vi "imp_test_v11_p3.vi"() -> ()   [LabVIEW 2014]
uses:
  <vilib>/LabVIEW Targets/FPGA/cRIO/shared/nicrio_ModuleControls/nicrio_cRIO-9237_DataRatesRing.ctl
  <vilib>/LabVIEW Targets/FPGA/cRIO/shared/nicrio_ModuleControls/nicrio_cRIO-9237_ExcitationVoltageRing.ctl
  <vilib>/rvi/FXPMathLib/FxpSinAndCos/subVIs/nifxpmath_SinAndCos_SimConfig.ctl
  <vilib>/rvi/Emulation/niFpgaGetClockAttributes.vi
  <vilib>/rvi/Emulation/niFpgaSctlEmulationGetInTimedLoop.vi
  <vilib>/rvi/Emulation/niFpgaEmulationReportErrorSimple.vi
  <vilib>/rvi/Emulation/niFpgaProcessEmulError.vi
  <vilib>/rvi/interface/RandomDataEmulation/nirviRandomDataMultiElementFPGAFIFO.vi
  <instcachedir>/0/nirviRandomDataMultiElementFPGAFIFO_AD0CFC12EF974623A9C2E4184BC062B2.lvgen/nirviRandomDataMultiElementFPGAFIFO_AD0CFC12EF974623A9C2E4184BC062B2_028.vi
  <vilib>/rvi/interface/RandomDataEmulation/niFpgaRandomDataHandleErrors.vi
  <vilib>/rvi/Emulation/niFpgaCriticalErrorInLSC.vi
  <vilib>/rvi/FXPMathLib/FxpSinAndCos/simVIs/DllFxpSinAndCosTemp_sub.vi
  <vilib>/rvi/eio/common/nirviEmuTemplateMethod_errors.vi
  <vilib>/rvi/eio/common/nirviEmuTemplatePropertySet_errors.vi
  <vilib>/rvi/DataTransferAndStorage/Container/XNode/niFpgaContainer.xnode
  <vilib>/rvi/interface/RandomDataEmulation/nirviRandomDataFpgaMultiElementTemplate.vi
  <vilib>/rvi/Analysis/measure/butterworth/XNode/niFpgaButterworthFilter.xnode
  <vilib>/rvi/FXPMathLib/FxpSinAndCos/XNode/nifxpmath_SinAndCos.xnode
  <vilib>/eio/EIONode/EIONode.xnode
  <vilib>/eio/EIOPropertyNode/EIOPropertyNode.xnode
  <vilib>/rvi/eio/common/nirviEmuTemplatePropertyGet_errors.vi
  <vilib>/rvi/eio/common/nirviEmuTemplatePropertyGet_noerrors.vi
  <vilib>/rvi/eio/common/nirviEmuTemplatePropertySet_noerrors.vi
panel:
  in  "force_lim":fxp<+,22,9>
  in  "Mavg f loop(uSec)":u32
  in  "F_Threshold_p":fxp<+,12,4>
  out "omega_p (Mavg)":fxp<+/-,36,13>
  out "Dp_d (Mavg)":fxp<+/-,36,13>
  out "omega_p2 (Mavg)":fxp<+/-,36,14>
  out "Dp2_d (Mavg)":fxp<+/-,36,14>
  in  "mt0_p2":u32
  out "Dp_d (Mavg w. f.)":fxp<+/-,36,14>
  in  "Dp_d (Mavg) coeff.":i32[](array[numeric])=[946630756, 63555534]
  out "omega_p (Mavg w. f)":fxp<+/-,36,14>
  in  "omega_P(Mavg) coeff.":i32[](array[numeric])=[946630756, 63555534]
  out "PID (kHz)":fxp<+/-,20,10>
  in  "Set 6":bool
  in  "Set 5":bool
  in  "Set 4":bool
  in  "Set 3":bool
  in  "Set 2":bool
  in  "Set 1":bool
  out "Dp1_d (T)":fxp<+/-,36,13>
  out "omega_p1 (T)":fxp<+/-,36,13>
  out "Dp2_d (T)":fxp<+/-,36,13>
  out "omega_p2 (T)":fxp<+/-,36,13>
  out "mt_omega_p2":u32
  out "Encoder Position_p2":i32
  out "D_p2":fxp<+/-,32,7>
  out "rad_p2":fxp<+/-,33,20>
  out "D_p1":fxp<+/-,32,7>
  out "rad_p1":fxp<+/-,33,20>
  out "Encoder Position_p1":i32
  out "Dp1_d (Mavg)":fxp<+/-,36,14>
  out "omega_p1 (Mavg)":fxp<+/-,36,14>
  in  "Dp_d_M_avg_Tc (uSec)":i32
  out "Dp_d (T)":fxp<+/-,36,13>
  out "omega_p (T)":fxp<+/-,36,13>
  in  "Vp. Est.":i16(ring) items=["T", "Mavg", "Mavg w. f."]
  in  "Mag. factor_p":fxp<+/-,20,3>
  in  "Mag. encoder_p":bool
  in  "Belt_out_p":fxp<+/-,7,7>
  in  "Belt_in_p":fxp<+/-,6,6>
  out "Fp_dc":fxp<+/-,32,10>
  in  "Zero_p":bool
  in  "mt0_p1":u32
  in  "Encoder reset":bool
  out "fpt_d":fxp<+/-,36,18>
  out "Dp_error_dd":fxp<+/-,36,16>
  out "Dp_error_d":fxp<+/-,33,8>
  in  "Dp_dd coeff.":i32[](array[numeric])=[946630756, 63555534]
  out "Dp_dd":fxp<+/-,36,25>
  out "dFp_PID":fxp<+/-,36,18>
  in  "dFp_PID coeff.":i32[](array[numeric])=[946630756, 63555534]
  out "fpt_i":fxp<+/-,34,18>
  in  "Bv_p":fxp<+/-,22,8>
  in  "Kv_p":fxp<+/-,26,7>
  out "Dp_error":fxp<+/-,22,7>
  out "Dpr_sin":fxp<+/-,22,7>
  in  "Sin offset_p":fxp<+/-,22,7>
  in  "Sin magnitude_p":fxp<+/-,21,6>
  out "Dpr_sin_dd":fxp<+/-,35,20>
  out "Dpr_sin_d":fxp<+/-,33,15>
  out "Sin omega_p":fxp<+/-,34,9>
  in  "Sin wave freq._p (Hz)":fxp<+/-,32,6>
  in  "Dpr_step":fxp<+/-,22,7>
  out "Dpr_for":fxp<+/-,22,7>
  in  "Command_p":i16(ring) items=["Step", "Sine"]
  in  "Ki_p":fxp<+/-,30,9>
  out "Fp_PID":fxp<+/-,36,16>
  in  "fp_tolorance":fxp<+,22,6>
  out "fp_tilde":fxp<+/-,33,10>
  in  "Kd_p":fxp<+/-,30,9>
  in  "Kp_p":fxp<+/-,32,13>
  out "Fr_p":fxp<+/-,32,10>
  in  "S/F coeff_p":fxp<+/-,25,-10>
  out "va_p":fxp<+/-,36,7>
  out "vb_p":fxp<+/-,37,8>
  out "vq_p_F":fxp<+/-,20,5> format="%.57g"
  out "vd_p_F":fxp<+/-,20,5>
  in  "dFp_add":bool
  in  "Stop motor_p":bool
  out "Force_p":fxp<+/-,32,10>
  in  "Strain selection_p":i16(ring) items=["Raw", "Avg.8", "Avg.8 w. filter"]
  out "Strain_p (Avg8 w. f)":fxp<+/-,36,8>
  in  "Strain_p Avg.8 coeff.":i32[](array[numeric])=[946630756, 63555534]
  out "Strain_p (Avg8)":fxp<+/-,36,4>
  out "Raw Strain_p":fxp<+/-,36,4>
  out "Mod6/AI3":fxp<+/-,36,4>
  in  "Strain gage reset_p":bool
  out "Dp_d (mm/s)":fxp<+/-,36,13>
  out "omega_p (rad/s)":fxp<+/-,36,13>
  out "mt_omega_p1":u32
  out "rad_p(NrTheta)":fxp<+/-,33,20>
  out "D_p(mm)":fxp<+/-,32,7>
  out "Encoder Position_p":i32
  in  "Encoder reset_p":bool
  out "Time now(s)":fxp<+,52,14>
  in  "Drive mode":i16(ring) items=["Backward", "Forward", "Imp"]
  in  "Ini coe.":bool
  out "Loop rate (kHz)":fxp<+/-,36,7>
  in  "Stop (Strain)":bool
  in  "Excitation Voltage":T1 items=["2.5 Volts", "3.3 Volts", "5.0 Volts", "10.0 Volts", "External Excitation"]
  in  "Data Rate":T2=1 items=["50.000 kS/s (NI 9237)"=1, "25.000 kS/s (NI 9237)"=2, "16.667 kS/s (NI 9237)"=3, "12.500 kS/s (NI 9237)"=4, "10.000 kS/s (NI 9237)"=5, "8.333 kS/s (NI 9237)"=6, "7.143 kS/s (NI 9237)"=7, "6.250 kS/s (NI 9237)"=8, "5.556 kS/s (NI 9237)"=9, "5.000 kS/s (NI 9237)"=10, "4.545 kS/s (NI 9237)"=11, "4.167 kS/s (NI 9237)"=12, "3.846 kS/s (NI 9237)"=13, "3.571 kS/s (NI 9237)"=14, "3.333 kS/s (NI 9237)"=15, "3.125 kS/s (NI 9237)"=16, "2.941 kS/s (NI 9237)"=17, "2.778 kS/s (NI 9237)"=18, "2.632 kS/s (NI 9237)"=19, "2.500 kS/s (NI 9237)"=20, "2.381 kS/s (NI 9237)"=21, "2.273 kS/s (NI 9237)"=22, "2.174 kS/s (NI 9237)"=23, "2.083 kS/s (NI 9237)"=24, "2.000 kS/s (NI 9237)"=25, "1.923 kS/s (NI 9237)"=26, "1.852 kS/s (NI 9237)"=27, "1.786 kS/s (NI 9237)"=28, "1.724 kS/s (NI 9237)"=29, "1.667 kS/s (NI 9237)"=30, "1.613 kS/s (NI 9237)"=31]
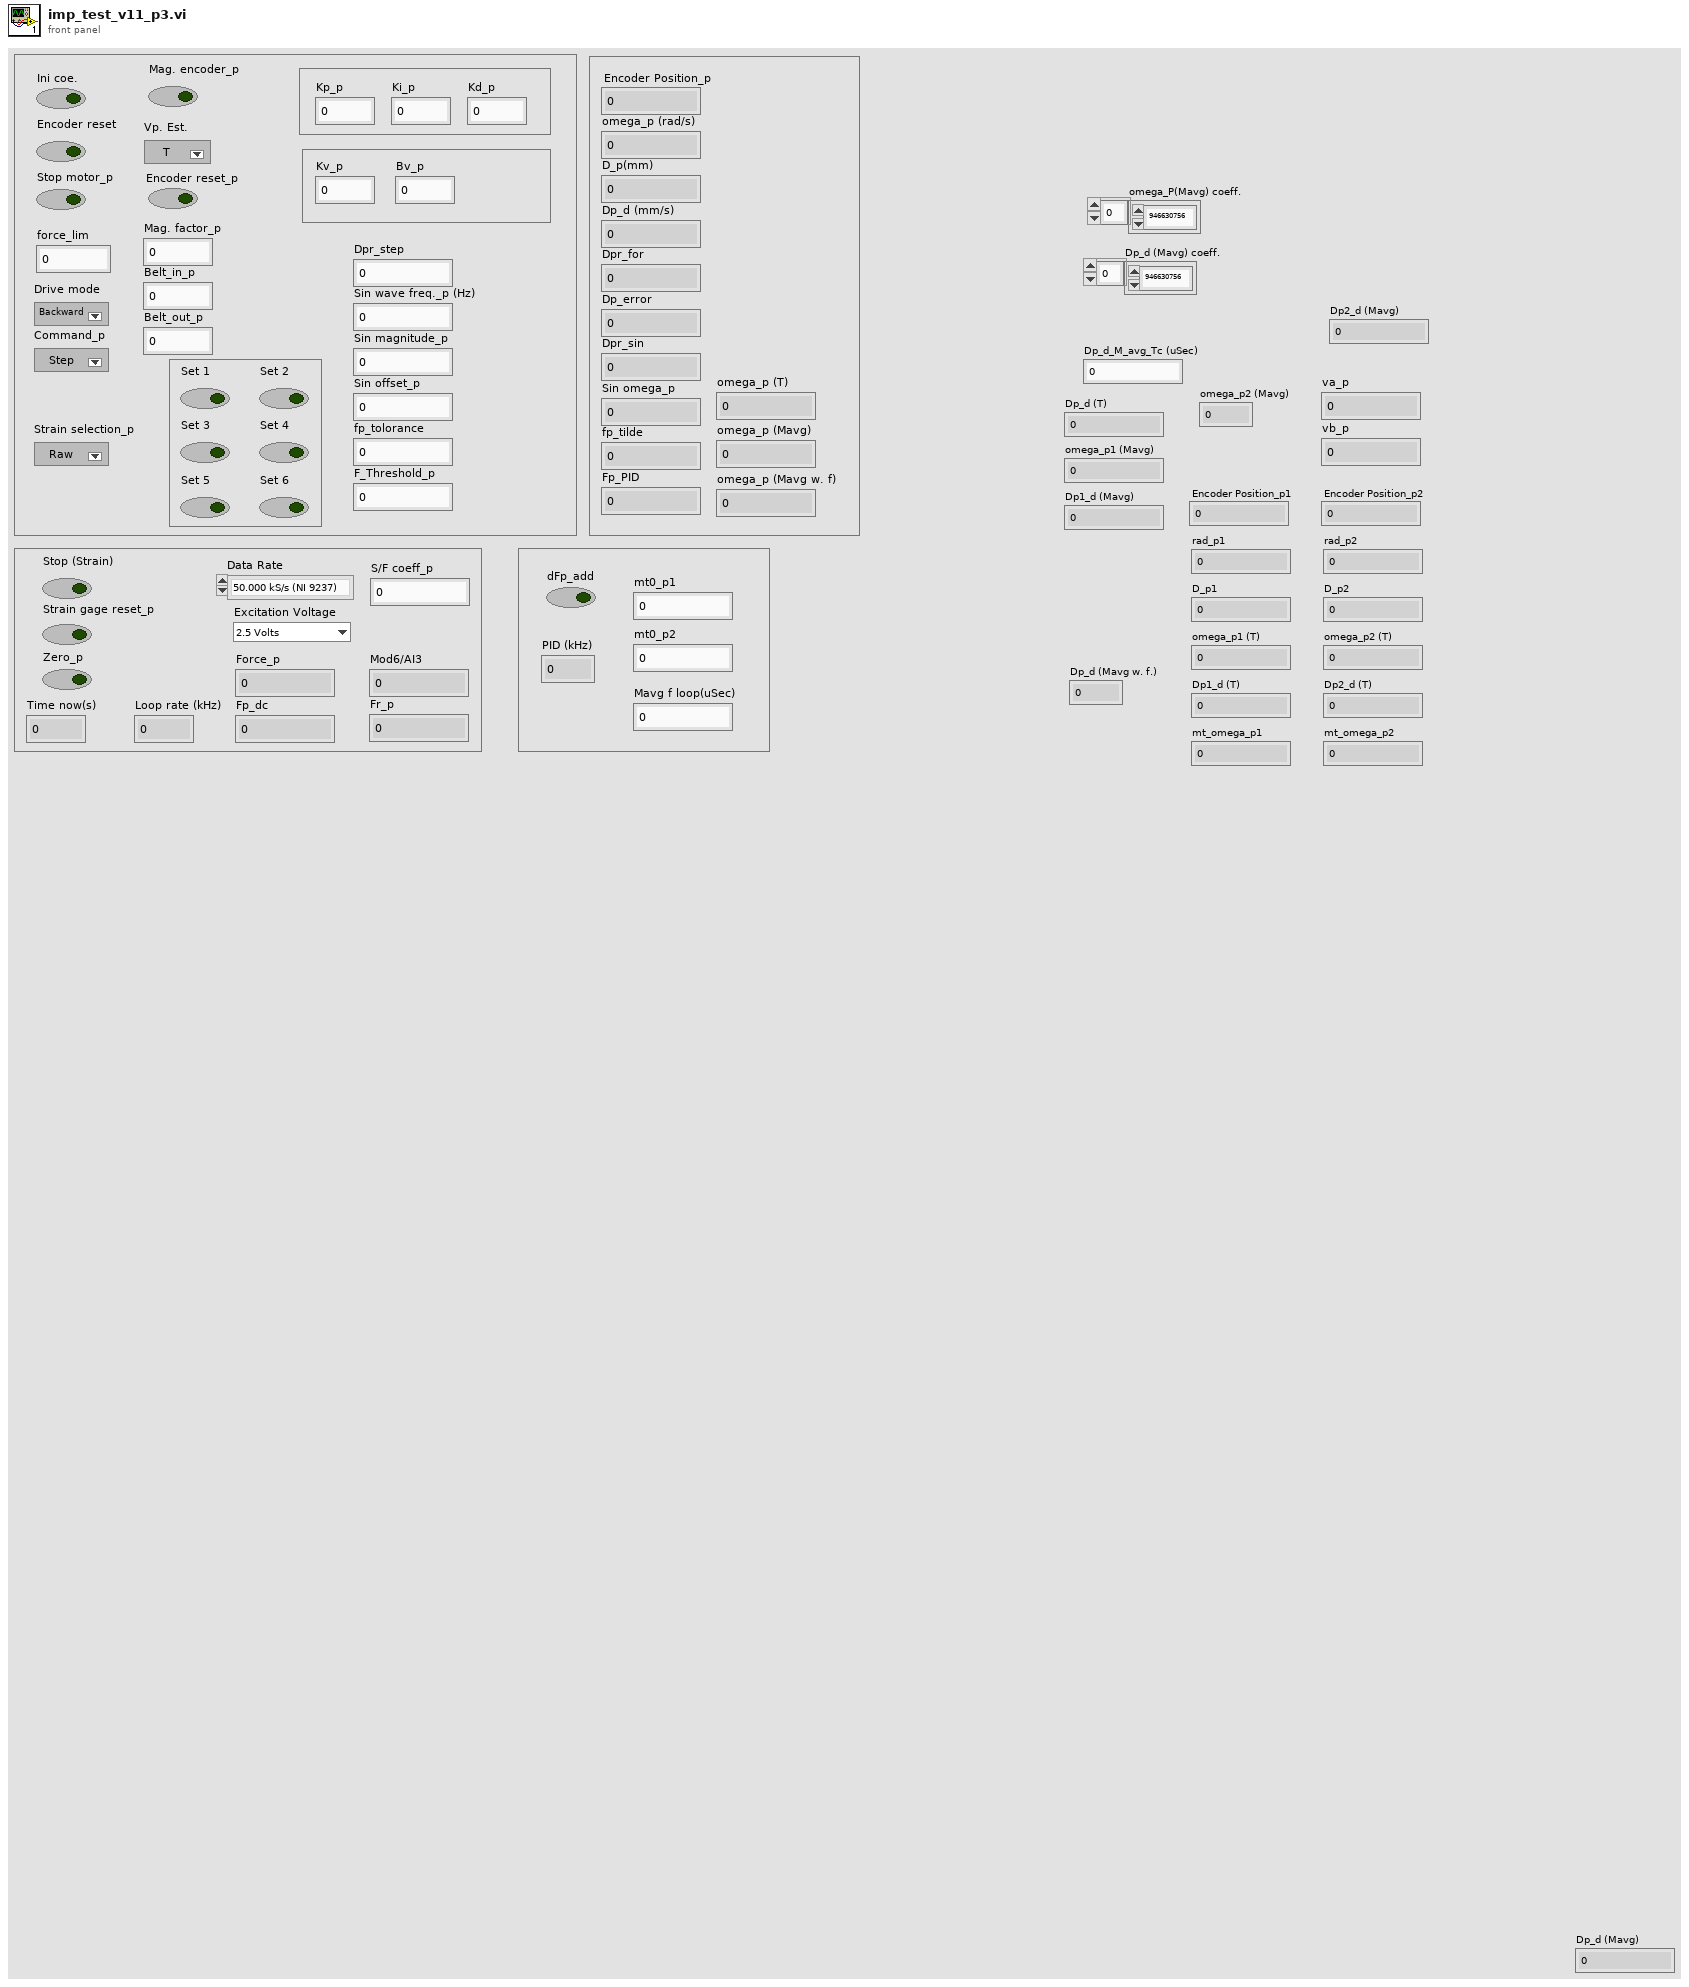
[diagram p1: front panel]
types:
  T1 = typedef "nicrio_cRIO-9237_ExcitationVoltageRing.ctl" = u8
  T2 = typedef "nicrio_cRIO-9237_DataRatesRing.ctl" = u8
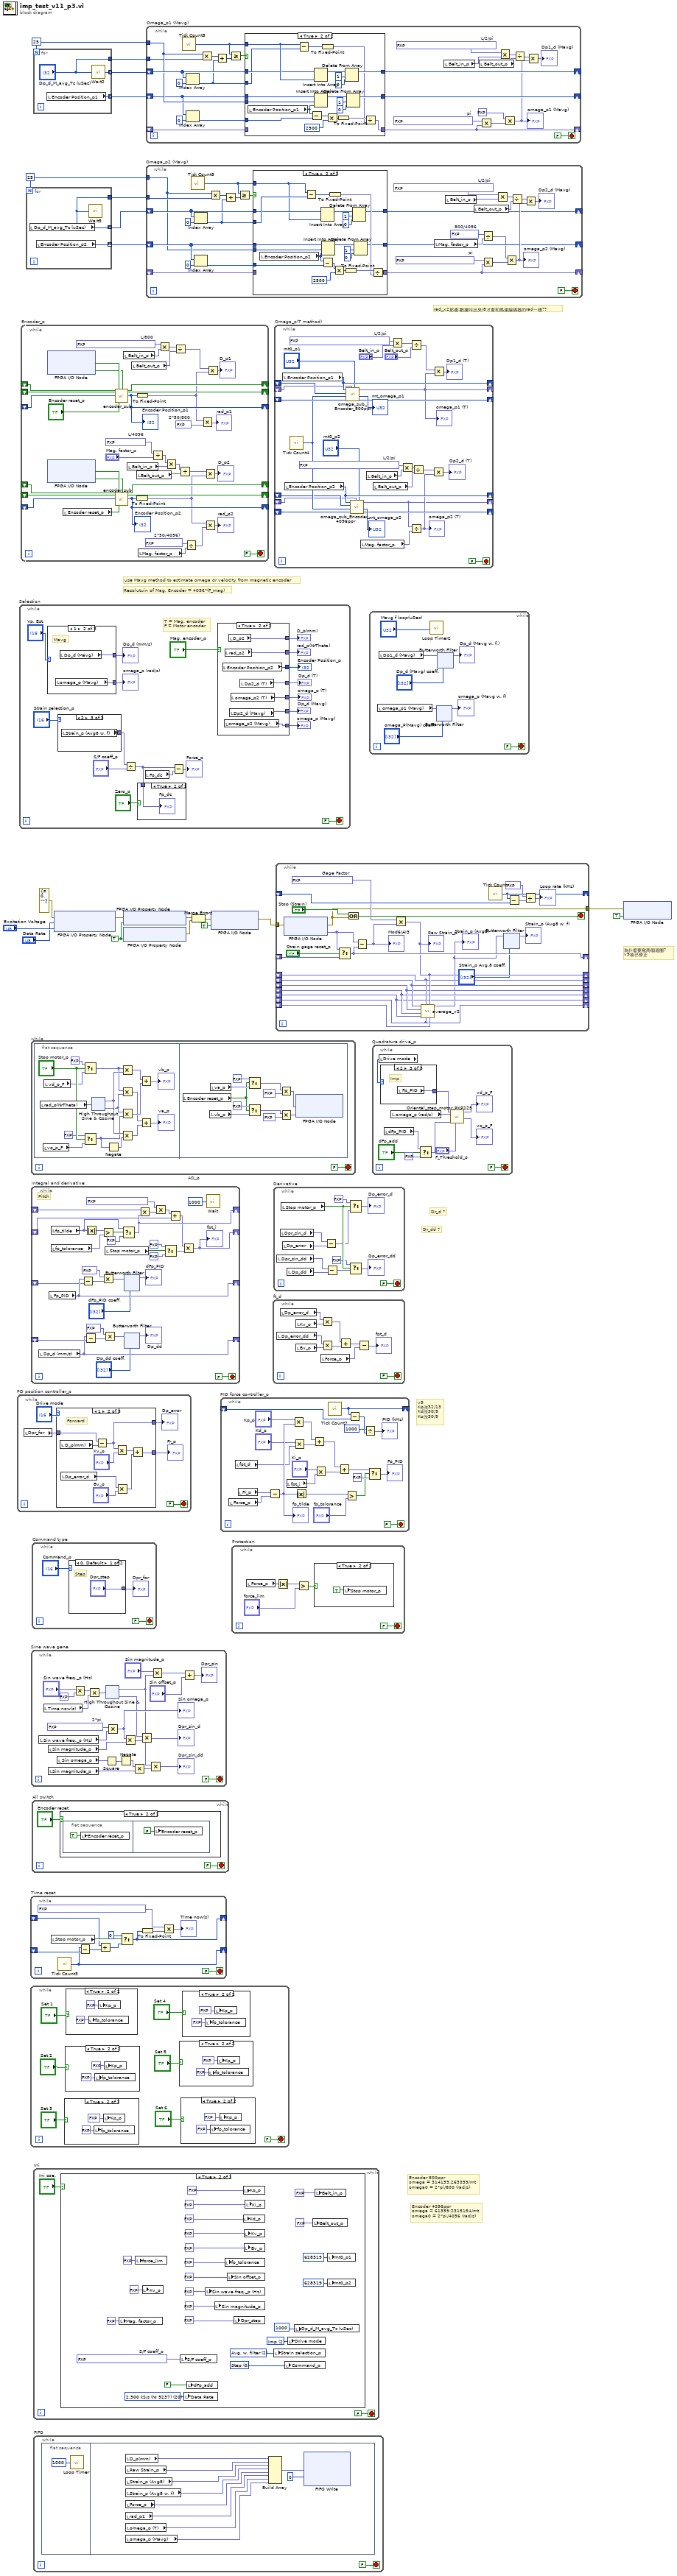
[diagram p0: block diagram]
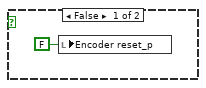
[diagram p11: hidden frame]
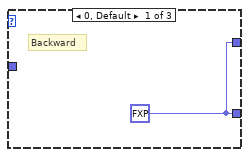
[diagram p12: hidden frame]
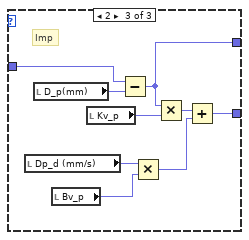
[diagram p13: hidden frame]
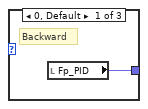
[diagram p14: hidden frame]
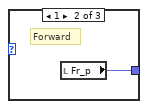
[diagram p15: hidden frame]
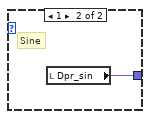
[diagram p16: hidden frame]
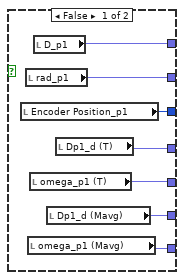
[diagram p17: hidden frame]
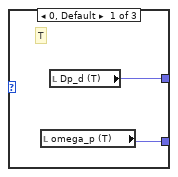
[diagram p18: hidden frame]
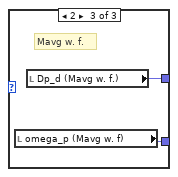
[diagram p19: hidden frame]
diagram:
  w2 = 25
  w8 = 25
  w13 = TRUE ("Half-Bridge Enable")
  # "rad_x2那邊:數據叫出來/8才會和馬達編碼器的rad一樣??"
  # "Encoder 4096ppr\nomega = 61359.2315154/mt\nomega0 = 2*pi/4096 (rad/s)"
  # "Encoder 800ppr\nomega = 314159.265359/mt\nomega0 = 2*pi/800 (rad/s)"
  # "v9\nKp改32/13\nKd改30/9\nKo改30/9"
  # "Resolutuin of Mag. Encoder = 4096*(F_mag)"
  # "use Mavg method to estimate omega or velocity from magnetic encoder"
  # "為什麼要寫兩個迴圈?\nv9後已修正"
  # "Dr_dd ?"
  # "Dr_d ?"
  n1 = while "PD position controller_p" {
    stop <- FALSE stop-if-true
    n2 = local read "Dpr_for"() -> (w21:fxp<+/-,22,7>)
    n3 = case shown="1" "Drive mode" {
      tunnel: [w26 w30 w37] -> w25
      tunnel: [w26 w28 w42] -> w22
      tunnel: w21 -> [_ w27 w36]
      frame 0, Default {
        w26 = fxp<+/-,62,19> 0.0
        # "Backward"
      }
      frame 1 {
        # "Forward"
        n4 = local read "D_p(mm)"() -> (w35:fxp<+/-,32,7>)
        n5 = local read "Dp_error_d"() -> (w29:fxp<+/-,33,8>)
        n6 = Subtract(x=w27, y=w35) -> (x-y=w28:fxp<+/-,33,8>)
        n7 = Multiply(x=w28, y="Kv_p") -> (x*y=w32:fxp<+/-,58,14>)
        n8 = Multiply(x=w29, y="Bv_p") -> (x*y=w31:fxp<+/-,55,16>)
        n9 = Add(x=w32, y=w31) -> (x+y=w30:fxp<+/-,60,16>)
      }
      frame 2 {
        # "Imp"
        n10 = local read "Dp_d (mm/s)"() -> (w40:fxp<+/-,36,13>)
        n11 = local read "D_p(mm)"() -> (w43:fxp<+/-,32,7>)
        n12 = local read "Bv_p"() -> (w39:fxp<+/-,22,8>)
        n13 = local read "Kv_p"() -> (w44:fxp<+/-,26,7>)
        n14 = Subtract(x=w36, y=w43) -> (x-y=w42:fxp<+/-,33,8>)
        n15 = Multiply(x=w40, y=w39) -> (x*y=w38:fxp<+/-,58,21>)
        n16 = Multiply(x=w42, y=w44) -> (x*y=w41:fxp<+/-,58,14>)
        n17 = Add(x=w41, y=w38) -> (x+y=w37:fxp<+/-,64,21>)
      }
    }
    "Fr_p" <- w25
    "Dp_error" <- w22
  }
  n18 = while "Selection" {
    stop <- FALSE stop-if-true
    # "T = Mag. encoder\nF = Motor encoder"
    n19 = case shown="1" "Vp. Est." {
      tunnel: [w79 w80 w83] -> w55
      tunnel: [w78 w81 w82] -> w56
      frame 0, Default {
        # "T"
        n20 = local read "omega_p (T)"() -> (w79:fxp<+/-,36,13>)
        n21 = local read "Dp_d (T)"() -> (w78:fxp<+/-,36,13>)
      }
      frame 1 {
        # "Mavg"
        n22 = local read "omega_p (Mavg)"() -> (w80:fxp<+/-,36,13>)
        n23 = local read "Dp_d (Mavg)"() -> (w81:fxp<+/-,36,13>)
      }
      frame 2 {
        # "Mavg w. f."
        n24 = local read "omega_p (Mavg w. f)"() -> (w83:fxp<+/-,36,14>)
        n25 = local read "Dp_d (Mavg w. f.)"() -> (w82:fxp<+/-,36,14>)
      }
    }
    "Dp_d (mm/s)" <- w56
    "omega_p (rad/s)" <- w55
    n26 = case shown="2" "Strain selection_p" {
      tunnel: [w85 w86 w87] -> w62
      frame 0, Default {
        n27 = local read "Raw Strain_p"() -> (w85:fxp<+/-,36,4>)
      }
      frame 1 {
        n28 = local read "Strain_p (Avg8)"() -> (w86:fxp<+/-,36,4>)
      }
      frame 2 {
        n29 = local read "Strain_p (Avg8 w. f)"() -> (w87:fxp<+/-,36,8>)
      }
    }
    n30 = Divide(x=w62, y="S/F coeff_p") -> (x/y=w59:fxp<+/-,32,10>)
    n31 = case shown="True" "Zero_p" {
      tunnel: w59 -> [_ w84]
      frame False {
      }
      frame True {
        "Fp_dc" <- w84
      }
    }
    n32 = local read "Fp_dc"() -> (w57:fxp<+/-,32,10>)
    n33 = Subtract(x=w59, y=w57) -> (x-y=→"Force_p":fxp<+/-,33,11>)
    n34 = case shown="True" "Mag. encoder_p" {
      tunnel: [w70 w77] -> w51
      tunnel: [w69 w76] -> w52
      tunnel: [w68 w75] -> w53
      tunnel: [w66 w74] -> w49
      tunnel: [w67 w73] -> w48
      tunnel: [w65 w71] -> w47
      tunnel: [w64 w72] -> w46
      frame False {
        n35 = local read "Encoder Position_p1"() -> (w68:i32)
        n36 = local read "rad_p1"() -> (w69:fxp<+/-,33,20>)
        n37 = local read "omega_p1 (Mavg)"() -> (w64:fxp<+/-,36,14>)
        n38 = local read "omega_p1 (T)"() -> (w66:fxp<+/-,36,13>)
        n39 = local read "D_p1"() -> (w70:fxp<+/-,32,7>)
        n40 = local read "Dp1_d (Mavg)"() -> (w65:fxp<+/-,36,14>)
        n41 = local read "Dp1_d (T)"() -> (w67:fxp<+/-,36,13>)
      }
      frame True {
        n42 = local read "Encoder Position_p2"() -> (w75:i32)
        n43 = local read "omega_p2 (Mavg)"() -> (w72:fxp<+/-,36,14>)
        n44 = local read "rad_p2"() -> (w76:fxp<+/-,33,20>)
        n45 = local read "D_p2"() -> (w77:fxp<+/-,32,7>)
        n46 = local read "Dp2_d (Mavg)"() -> (w71:fxp<+/-,36,14>)
        n47 = local read "omega_p2 (T)"() -> (w74:fxp<+/-,36,13>)
        n48 = local read "Dp2_d (T)"() -> (w73:fxp<+/-,36,13>)
      }
    }
    "D_p(mm)" <- w51
    "rad_p(NrTheta)" <- w52
    "Encoder Position_p" <- w53
    "Dp_d (T)" <- w48
    "omega_p (T)" <- w49
    "Dp_d (Mavg)" <- w47
    "omega_p (Mavg)" <- w46
  }
  n49 = while "Encoder_p" {
    shift-right: [w125] -> _
    shift-left: _ -> [w124]
    shift-right: [w126] -> _
    shift-left: _ -> [w123]
    shift-right: [w120] -> _
    shift-left: _ -> [w122]
    shift-right: [w111] -> _
    shift-left: _ -> [w110]
    shift-right: [w112] -> _
    shift-left: _ -> [w113]
    shift-right: [w107] -> _
    shift-left: _ -> [w108]
    stop <- FALSE stop-if-true
    w103 = fxp<+/-,20,-5> 0.00048828125  # L/4096
    w101 = fxp<+/-,16,1> 0.0244140625  # 2*50/4096)
    w119 = fxp<+/-,20,-5> 0.002499997615814209  # L/800
    w93 = fxp<+/-,16,1> 0.125  # 2*50/800
    n50 = xnode "FPGA I/O Node"() -> ("Mod7/DIO0"=w128:bool, "Mod7/DIO1"=w127:bool)  [unwired: 2 in, 2 out]
    n51 = xnode "FPGA I/O Node"() -> ("Mod7/DIO4"=w115:bool, "Mod7/DIO5"=w114:bool)  [unwired: 2 in, 2 out]
    n52 = local read "Encoder reset_p"() -> (w109:bool)
    n53 = call "encoder_sub.vi"("A_pre"=w124, "B_pre"=w123, "Encoder Position_pre"=w122, "A input"=w128, "Encoder Position Reset"="Encoder reset_p", "B input"=w127) -> ("A"=w125:bool, "B"=w126:bool, "Encoder Position (Counts)"=w120:i32)  [unwired: 19 in]
    "Encoder Position_p1" <- w120
    n54 = call "encoder_sub.vi"("A_pre"=w110, "B_pre"=w113, "Encoder Position_pre"=w108, "A input"=w115, "Encoder Position Reset"=w109, "B input"=w114) -> ("A"=w111:bool, "B"=w112:bool, "Encoder Position (Counts)"=w107:i32)  [unwired: 19 in]
    "Encoder Position_p2" <- w107
    n55 = local read "Belt_in_p"() -> (w118:fxp<+/-,6,6>)
    n56 = local read "Belt_in_p"() -> (w104:fxp<+/-,6,6>)
    n57 = local read "Belt_out_p"() -> (w116:fxp<+/-,7,7>)
    n58 = To Fixed-Point(number=w107) -> (fixed-point=w89:fxp<+/-,32,32>)  [unwired: 1 in]
    n59 = To Fixed-Point(number=w120) -> (fixed-point=w94:fxp<+/-,32,32>)  [unwired: 1 in]
    n60 = local read "Belt_out_p"() -> (w106:fxp<+/-,7,7>)
    n61 = local read "Mag. factor_p"() -> (w100:fxp<+/-,20,3>)
    n62 = Divide(x=w103, y="Mag. factor_p") -> (x/y=w102:fxp<+/-,41,13>)
    n63 = Multiply(x=w119, y=w118) -> (x*y=w117:fxp<+/-,26,1>)
    n64 = Multiply(x=w102, y=w104) -> (x*y=w105:fxp<+/-,46,18>)
    n65 = Divide(x=w117, y=w116) -> (x/y=w96:fxp<+/-,33,1>)
    n66 = Divide(x=w105, y=w106) -> (x/y=w91:fxp<+/-,53,18>)
    n67 = Divide(x=w101, y=w100) -> (x/y=w88:fxp<+/-,37,5>)
    n68 = Multiply(x=w94, y=w93) -> (x*y=→"rad_p1":fxp<+/-,33,20>)
    n69 = Multiply(x=w91, y=w89) -> (x*y=→"D_p2":fxp<+/-,37,7>)
    n70 = Multiply(x=w89, y=w88) -> (x*y=→"rad_p2":fxp<+/-,46,16>)
    n71 = Multiply(x=w96, y=w94) -> (x*y=→"D_p1":fxp<+/-,32,7>)
  }
  n72 = for {
    N: w2 -> [_]
    tunnel: [w130] -> w4 mode=indexing
    tunnel: [w129] -> w3 mode=indexing
    tunnel: [w129] -> w1
    n73 = local read "Dp_d_M_avg_Tc (uSec)"() -> (w129:i32)
    n74 = local read "Encoder Position_p2"() -> (w130:i32)
    n75 = call "Wait5"("Count(uSec)"=w129) -> ()  [unwired: 1 out]
  }
  n76 = while "Time reset" {
    shift-right: [w140] -> _
    shift-left: _ -> [w141]
    shift-right: [w135] -> _
    shift-left: _ -> [w136]
    stop <- FALSE stop-if-true
    n77 = local read "Stop motor_p"() -> (w142:bool)
    n78 = call "Tick Count3"() -> ("Tick Count(uSec)"=w140:u32)
    n79 = Subtract(x=w140, y=w141) -> (x-y=w139:u32)
    n80 = Add(x=w136, y=w139) -> (x+y=w138:u32)
    n81 = Select(t=u32 0, s=w142, f=w138) -> (s? t:f=w135:u32)
    n82 = To Fixed-Point(number=w135) -> (fixed-point=w134:fxp<+,32,32>)  [unwired: 1 in]
    n83 = Multiply(x=fxp<+,20,-18> 1.0000003385357559e-06, y=w134) -> (x*y=→"Time now(s)":fxp<+,52,14>)
  }
  n84 = while {
    stop <- FALSE stop-if-true
    n85 = case shown="True" "Set 3" {
      frame False {
      }
      frame True {
        n86 = local write "fp_tolorance"(fxp<+,22,6> 3.0 ("fp_tolorance")) -> ()
        n87 = local write "Kp_p"(fxp<+/-,36,9> 100.0 ("Kp_p")) -> ()
      }
    }
    n88 = case shown="True" "Set 2" {
      frame False {
      }
      frame True {
        n89 = local write "fp_tolorance"(fxp<+,22,6> 1.5 ("fp_tolorance")) -> ()
        n90 = local write "Kp_p"(fxp<+/-,36,9> 50.0 ("Kp_p")) -> ()
      }
    }
    n91 = case shown="True" "Set 1" {
      frame False {
      }
      frame True {
        n92 = local write "fp_tolorance"(fxp<+,22,6> 3.0 ("fp_tolorance")) -> ()
        n93 = local write "Kp_p"(fxp<+/-,36,9> 50.0 ("Kp_p")) -> ()
      }
    }
    n94 = case shown="True" "Set 5" {
      frame False {
      }
      frame True {
        n95 = local write "fp_tolorance"(fxp<+,22,6> 3.0 ("fp_tolorance")) -> ()
        n96 = local write "Kp_p"(fxp<+/-,36,9> 150.0 ("Kp_p")) -> ()
      }
    }
    n97 = case shown="True" "Set 6" {
      frame False {
      }
      frame True {
        n98 = local write "fp_tolorance"(fxp<+,22,6> 1.5 ("fp_tolorance")) -> ()
        n99 = local write "Kp_p"(fxp<+/-,36,9> 150.0 ("Kp_p")) -> ()
      }
    }
    n100 = case shown="True" "Set 4" {
      frame False {
      }
      frame True {
        n101 = local write "fp_tolorance"(fxp<+,22,6> 1.5 ("fp_tolorance")) -> ()
        n102 = local write "Kp_p"(fxp<+/-,36,9> 100.0 ("Kp_p")) -> ()
      }
    }
  }
  n103 = while "AO_p" {
    stop <- FALSE stop-if-true
    n104 = flat-sequence {
      frame #0 {
        n105 = local read "rad_p(NrTheta)"() -> (w174:fxp<+/-,33,20>)
        n106 = local read "vq_p_F"() -> (w175:fxp<+/-,20,5>)
        n107 = local read "vd_p_F"() -> (w177:fxp<+/-,20,5>)
        n108 = Select(t=fxp<+/-,20,5> 0.0, s="Stop motor_p", f=w177) -> (s? t:f=w166:fxp<+/-,20,5>)
        n109 = Select(t=fxp<+,1,1> 0.0, s="Stop motor_p", f=w175) -> (s? t:f=w165:fxp<+/-,20,5>)
        n110 = xnode "High Throughput Sine & Cosine"("x (pi)"=w174) -> ("sin(x)"=w168:fxp<+/-,16,2>, "cos(x)"=w167:fxp<+/-,16,2>)
        n111 = Negate(x=w165) -> (-x=w173:fxp<+/-,21,6>)
        n112 = Multiply(x=w166, y=w168) -> (x*y=w172:fxp<+/-,36,7>)
        n113 = Multiply(x=w166, y=w167) -> (x*y=w170:fxp<+/-,36,7>)
        n114 = Multiply(x=w167, y=w165) -> (x*y=w171:fxp<+/-,36,7>)
        n115 = Multiply(x=w168, y=w173) -> (x*y=w169:fxp<+/-,35,6>)
        n116 = Add(x=w172, y=w171) -> (x+y=→"vb_p":fxp<+/-,37,8>)
        n117 = Add(x=w170, y=w169) -> (x+y=→"va_p":fxp<+/-,36,7>)
      }
      frame #1 {
        n118 = local read "Encoder reset_p"() -> (w210:bool)
        n119 = local read "vb_p"() -> (w211:fxp<+/-,37,8>)
        n120 = local read "va_p"() -> (w212:fxp<+/-,36,7>)
        n121 = Select(t=fxp<+,2,2> 3.0, s=w210, f=w212) -> (s? t:f=w218:fxp<+/-,36,7>)
        n122 = Select(t=fxp<+,1,1> 0.0, s=w210, f=w211) -> (s? t:f=w217:fxp<+/-,37,8>)
        n123 = Multiply(x=w218, y=fxp<+/-,1,0> -0.5) -> (x*y=w213:fxp<+/-,36,6>)
        n124 = Multiply(x=w217, y=fxp<+/-,1,0> -0.5) -> (x*y=w214:fxp<+/-,36,6>)
        n125 = xnode "FPGA I/O Node"("Mod8/AO0"=w213, "Mod8/AO1"=w214) -> ()  [unwired: 2 in, 2 out]
      }
    }
  }
  n126 = while "Sine wave gene" {
    stop <- FALSE stop-if-true
    w226 = fxp<+,20,3> 6.2831878662109375  # 2*pi
    n127 = local read "Sin wave freq._p (Hz)"() -> (w222:fxp<+/-,32,6>)
    n128 = local read "Time now(s)"() -> (w240:fxp<+,52,14>)
    n129 = local read "Sin magnitude_p"() -> (w223:fxp<+/-,21,6>)
    n130 = local read "Sin magnitude_p"() -> (w225:fxp<+/-,21,6>)
    n131 = local read "Sin omega_p"() -> (w224:fxp<+/-,34,9>)
    n132 = Multiply(x="Sin wave freq._p (Hz)", y=fxp<+/-,10,3> 2.0) -> (x*y=w244:fxp<+/-,42,9>)
    n133 = Multiply(x=w244, y=w240) -> (x*y=w241:fxp<+/-,41,19>)
    n134 = Square(x=w224) -> (x^2=w236:fxp<+,34,18>)
    n135 = xnode "High Throughput Sine & Cosine"("x (pi)"=w241) -> ("sin(x)"=w227:fxp<+/-,16,2>, "cos(x)"=w232:fxp<+/-,16,2>)
    n136 = Multiply(x=w226, y=w222) -> (x*y=w239:fxp<+/-,34,9>)
    "Sin omega_p" <- w239
    n137 = Negate(x=w236) -> (-x=w235:fxp<+/-,35,19>)
    n138 = Multiply(x=w239, y=w223) -> (x*y=w238:fxp<+/-,33,15>)
    n139 = Multiply(x=w235, y=w225) -> (x*y=w234:fxp<+/-,35,19>)
    n140 = Multiply(x=w232, y=w238) -> (x*y=→"Dpr_sin_d":fxp<+/-,33,15>)
    n141 = Multiply(x=w227, y=w234) -> (x*y=→"Dpr_sin_dd":fxp<+/-,35,20>)
    n142 = Multiply(x="Sin magnitude_p", y=w227) -> (x*y=w230:fxp<+/-,37,8>)
    n143 = Add(x=w230, y="Sin offset_p") -> (x+y=→"Dpr_sin":fxp<+/-,37,8>)
  }
  n144 = while "Integral and derivative" {
    shift-right: [w298] -> _
    shift-left: _ -> [w301]
    shift-right: [w291] -> _
    shift-left: _ -> [w290]
    shift-right: [w285] -> _
    shift-left: _ -> [w284]
    shift-right: [w280] -> _
    shift-left: _ -> [w281]
    stop <- FALSE stop-if-true
    # "Pitch"
    n145 = local read "Dp_d (mm/s)"() -> (w280:fxp<+/-,36,13>)
    n146 = local read "Fp_PID"() -> (w285:fxp<+/-,36,16>)
    n147 = local read "fp_tilde"() -> (w302:fxp<+/-,33,10>)
    n148 = local read "fp_tolorance"() -> (w305:fxp<+,22,6>)
    n149 = Subtract(x=w285, y=w284) -> (x-y=w289:fxp<+/-,37,17>)
    n150 = Subtract(x=w280, y=w281) -> (x-y=w282:fxp<+/-,37,14>)
    n151 = Absolute Value(x=w302) -> (abs(x)=w306:fxp<+,33,10>)
    n152 = Greater?(x=w306, y=w305) -> (0:w304:bool)
    n153 = Multiply(x=fxp<+,7,10> 1000.0, y=w289) -> (x*y=w287:fxp<+/-,32,18>)
    n154 = Multiply(x=fxp<+,7,10> 1000.0, y=w282) -> (x*y=w278:fxp<+/-,36,21>)
    n155 = local read "Stop motor_p"() -> (w293:bool)
    n156 = Select(t=w302, s=w304, f=fxp<+,1,1> 0.0) -> (s? t:f=w298:fxp<+/-,33,10>)
    n157 = xnode "Butterworth Filter"("input data"=w287, "scaled coefficients"="dFp_PID coeff.") -> ("output data"=→"dFp_PID":fxp<+/-,36,22>)  [unwired: 1 in]
    n158 = xnode "Butterworth Filter"("input data"=w278, "scaled coefficients"="Dp_dd coeff.") -> ("output data"=→"Dp_dd":fxp<+/-,36,25>)  [unwired: 1 in]
    n159 = Multiply(x=w301, y=w298) -> (x*y=w300:fxp<+/-,34,12>)
    n160 = Multiply(x=fxp<+/-,30,12> 0.000499725341796875, y=w300) -> (x*y=w297:fxp<+/-,34,10>)
    n161 = Select(t=fxp<+,1,1> 0.0, s=w293, f=fxp<+,1,1> 1.0) -> (s? t:f=w295:fxp<+,1,1>)
    n162 = Add(x=w297, y=w290) -> (x+y=w296:fxp<+/-,36,16>)
    n163 = Multiply(x=w296, y=w295) -> (x*y=w291:fxp<+/-,34,18>)
    "fpt_i" <- w291
    n164 = call "Wait"("Count(uSec)"=u32 1000) -> ()  [unwired: 1 out]
  }
  n165 = while "Command type" {
    stop <- FALSE stop-if-true
    n166 = case shown="0, Default" "Command_p" {
      tunnel: ["Dpr_step" w328] -> w325
      frame 0, Default {
        # "Step"
      }
      frame 1 {
        # "Sine"
        n167 = local read "Dpr_sin"() -> (w328:fxp<+/-,22,7>)
      }
    }
    "Dpr_for" <- w325
  }
  n168 = while "All switch" {
    stop <- FALSE stop-if-true
    n169 = case shown="True" "Encoder reset" {
      frame False {
        n170 = local write "Encoder reset_p"(FALSE ("Encoder reset_p")) -> ()
      }
      frame True {
        n171 = flat-sequence {
          frame #0 {
            n172 = local write "Encoder reset_p"(TRUE ("Encoder reset_p")) -> ()
          }
          frame #1 {
            n173 = local write "Encoder reset_p"(FALSE ("Encoder reset_p")) -> ()
          }
        }
      }
    }
  }
  n174 = for {
    N: w8 -> [_]
    tunnel: ["Dp_d_M_avg_Tc (uSec)"] -> w5
    tunnel: [w335] -> w7 mode=indexing
    tunnel: [w334] -> w6 mode=indexing
    n175 = local read "Encoder Position_p1"() -> (w334:i32)
    n176 = call "Wait2"("Count(uSec)"="Dp_d_M_avg_Tc (uSec)") -> ("Tick Count(uSec)"=w335:u32)
  }
  n177 = while "Ini" {
    stop <- FALSE stop-if-true
    n178 = case shown="True" "Ini coe." {
      frame False {
      }
      frame True {
        w341 = i16 2 items=["Backward", "Forward", "Imp"] ("Drive mode")
        w345 = T2 20 items=["50.000 kS/s (NI 9237)"=1, "25.000 kS/s (NI 9237)"=2, "16.667 kS/s (NI 9237)"=3, "12.500 kS/s (NI 9237)"=4, "10.000 kS/s (NI 9237)"=5, "8.333 kS/s (NI 9237)"=6, "7.143 kS/s (NI 9237)"=7, "6.250 kS/s (NI 9237)"=8, "5.556 kS/s (NI 9237)"=9, "5.000 kS/s (NI 9237)"=10, "4.545 kS/s (NI 9237)"=11, "4.167 kS/s (NI 9237)"=12, "3.846 kS/s (NI 9237)"=13, "3.571 kS/s (NI 9237)"=14, "3.333 kS/s (NI 9237)"=15, "3.125 kS/s (NI 9237)"=16, "2.941 kS/s (NI 9237)"=17, "2.778 kS/s (NI 9237)"=18, "2.632 kS/s (NI 9237)"=19, "2.500 kS/s (NI 9237)"=20, "2.381 kS/s (NI 9237)"=21, "2.273 kS/s (NI 9237)"=22, "2.174 kS/s (NI 9237)"=23, "2.083 kS/s (NI 9237)"=24, "2.000 kS/s (NI 9237)"=25, "1.923 kS/s (NI 9237)"=26, "1.852 kS/s (NI 9237)"=27, "1.786 kS/s (NI 9237)"=28, "1.724 kS/s (NI 9237)"=29, "1.667 kS/s (NI 9237)"=30, "1.613 kS/s (NI 9237)"=31] ("Data Rate")
        w360 = i16 0 items=["Step", "Sine"] ("Command_p")
        w361 = i16 2 items=["Raw", "Avg.", "Avg. w. filter"] ("Strain selection_p")
        w362 = fxp<+/-,25,-10> 5.851034075021744e-07  # S/F coeff_p
        n179 = local write "Mag. factor_p"(fxp<+/-,20,3> 1.0 ("Mag. factor_p")) -> ()
        n180 = local write "force_lim"(fxp<+,32,10> 50.0 ("force_lim")) -> ()
        n181 = local write "Kv_p"(fxp<+/-,26,7> 1.0 ("Kv_p")) -> ()
        n182 = local write "S/F coeff_p"(w362) -> ()
        n183 = local write "Data Rate"(w345) -> ()
        n184 = local write "dFp_add"(FALSE ("dFp_add")) -> ()
        n185 = local write "Sin wave freq._p (Hz)"(fxp<+/-,32,6> 1.0 ("Sin wave freq._p (Hz)")) -> ()
        n186 = local write "Sin magnitude_p"(fxp<+/-,21,6> 5.0 ("Sin magnitude_p")) -> ()
        n187 = local write "fp_tolorance"(fxp<+,22,6> 5.0 ("fp_tolorance")) -> ()
        n188 = local write "Sin offset_p"(fxp<+/-,22,7> 0.0 ("Sin offset_p")) -> ()
        n189 = local write "Dpr_step"(fxp<+/-,22,7> 0.0 ("Dpr_step")) -> ()
        n190 = local write "Kp_p"(fxp<+/-,36,9> 30.0 ("Kp_p")) -> ()
        n191 = local write "Kd_p"(fxp<+/-,36,9> 0.0 ("Kd_p")) -> ()
        n192 = local write "Kv_p"(fxp<+/-,22,8> 0.0 ("Kv_p")) -> ()
        n193 = local write "Bv_p"(fxp<+/-,22,8> 0.0 ("Bv_p")) -> ()
        n194 = local write "Ki_p"(fxp<+/-,36,9> 0.0 ("Ki_p")) -> ()
        n195 = local write "Strain selection_p"(w361) -> ()
        n196 = local write "Command_p"(w360) -> ()
        n197 = local write "Drive mode"(w341) -> ()
        n198 = local write "Dp_d_M_avg_Tc (uSec)"(u32 1000 ("D_d_M_avg_Tc (uSec)")) -> ()
        n199 = local write "Belt_out_p"(fxp<+/-,7,7> 36.0 ("Belt_op")) -> ()
        n200 = local write "Belt_in_p"(fxp<+/-,6,6> 16.0 ("Belt_mp")) -> ()
        n201 = local write "mt0_p1"(u32 628319 ("mt0_p1")) -> ()
        n202 = local write "mt0_p2"(u32 628319 ("mt0_p2")) -> ()
      }
    }
  }
  n203 = while "FIFO" {
    stop <- FALSE stop-if-true
    n204 = flat-sequence {
      frame #0 {
        n205 = call "Loop Timer"("Count(uSec)"=u32 1000) -> ()  [unwired: 1 out]
      }
      frame #1 {
        n206 = local read "D_p(mm)"() -> (w372:fxp<+/-,32,7>)
        n207 = local read "Raw Strain_p"() -> (w371:fxp<+/-,36,4>)
        n208 = local read "Strain_p (Avg8)"() -> (w370:fxp<+/-,36,4>)
        n209 = local read "Strain_p (Avg8 w. f)"() -> (w369:fxp<+/-,36,8>)
        n210 = local read "Force_p"() -> (w368:fxp<+/-,32,10>)
        n211 = local read "rad_p1"() -> (w367:fxp<+/-,33,20>)
        n212 = local read "omega_p (T)"() -> (w366:fxp<+/-,36,13>)
        n213 = local read "omega_p (Mavg)"() -> (w365:fxp<+/-,36,13>)
        n214 = Build Array(w372, w371, w370, w369, w368, w367, w366, w365) -> (w373:fxp<+/-,52,20>[])
        n215 = xnode ("FIFO Write")("Element"=w373, "Timeout"=0) -> ()  [unwired: 1 in, 2 out]
      }
    }
  }
  n216 = xnode "FPGA I/O Property Node"("error in"=errorcluster {"status"=FALSE, "code"=0, "source"=""}, "Data Rate"="Data Rate", "Excitation Voltage"="Excitation Voltage") -> ("error out"=w18:errorcluster)  [unwired: 1 in, 1 out]
  n217 = xnode "FPGA I/O Property Node"("error in"=w18, "Half-Bridge Enable"=w13) -> ("error out"=w11:errorcluster)  [unwired: 1 in, 1 out]
  n218 = xnode "FPGA I/O Property Node"("Half-Bridge Enable"=w13) -> ("error out"=w10:errorcluster)  [unwired: 2 in, 1 out]
  n219 = while "Omega_p2 (Mavg)" {
    shift-right: [w376] -> _
    shift-left: w4 -> [w397]
    shift-right: [w377] -> _
    shift-left: w3 -> [w395]
    shift-right: [w381] -> _
    shift-left: _ -> [w379]
    tunnel: w2 -> [w393]
    tunnel: w1 -> [w398]
    stop <- FALSE stop-if-true
    w382 = fxp<+/-,27,3> 3.1415926814079285  # pi
    w385 = fxp<+,32,0> 0.1953125  # 800/4096
    w390 = fxp<+/-,32,0> 0.3183098859153688  # L/2/pi
    n220 = call "Tick Count9"() -> ("Tick Count(uSec)"=w392:u32)
    n221 = Index Array(array=w395, index=0) -> (element=w394:i32)
    n222 = Index Array(array=w397, index=0) -> (element=w396:i32)
    n223 = Multiply(x=w393, y=w398) -> (x*y=w401:i32)
    n224 = Add(x=w401, y=w394) -> (x+y=w400:i32)
    n225 = Greater Or Equal?(x=w392, y=w400) -> (x >= y?=w399:bool)
    n226 = case shown="True" w399 {
      tunnel: w397 -> [w405 w420]
      tunnel: w396 -> [_ w412]
      tunnel: w395 -> [w406 w421]
      tunnel: w394 -> [_ w422]
      tunnel: w393 -> [_ w419]
      tunnel: w392 -> [_ w407]
      tunnel: [w405 w410] -> w376
      tunnel: [w406 w409] -> w377
      tunnel: [w404 w408] -> w381
      tunnel: w379 -> [w404 _]
      frame False {
      }
      frame True {
        n227 = local read "Encoder Position_p2"() -> (w411:i32)
        n228 = Subtract(x=w407, y=w422) -> (x-y=w423:u32)
        n229 = Insert Into Array(array=w421, new element=w407) -> (w425:i32[])  [unwired: 1 in]
        n230 = Subtract(x=w411, y=w412) -> (x-y=w416:i32)
        n231 = Insert Into Array(array=w420, index=w419, new element=w411) -> (w426:i32[])
        n232 = To Fixed-Point(number=w423) -> (fixed-point=w413:fxp<+,32,32>)  [unwired: 1 in]
        n233 = Multiply(x=w416, y=2500) -> (x*y=w417:i32)
        n234 = To Fixed-Point(number=w417) -> (fixed-point=w418:fxp<+/-,32,32>)  [unwired: 1 in]
        n235 = Delete From Array(array=w425, length=1, index=0) -> (array with subset deleted=w409:i32[])  [unwired: 1 out]
        n236 = Delete From Array(array=w426, length=1, index=0) -> (array with subset deleted=w410:i32[])  [unwired: 1 out]
        n237 = Divide(x=w418, y=w413) -> (x/y=w408:fxp<+/-,64,32>)
      }
    }
    n238 = local read "Mag. factor_p"() -> (w384:fxp<+/-,20,3>)
    n239 = local read "Belt_in_p"() -> (w387:fxp<+/-,6,6>)
    n240 = local read "Belt_out_p"() -> (w386:fxp<+/-,7,7>)
    n241 = Divide(x=w385, y=w384) -> (x/y=w375:fxp<+/-,32,1>)
    n242 = Multiply(x=w382, y=w381) -> (x*y=w383:fxp<+/-,64,35>)
    n243 = Multiply(x=w390, y=w387) -> (x*y=w391:fxp<+/-,38,6>)
    n244 = Multiply(x=w375, y=w383) -> (x*y=w378:fxp<+/-,64,36>)
    "omega_p2 (Mavg)" <- w378
    n245 = Divide(x=w391, y=w386) -> (x/y=w389:fxp<+/-,45,6>)
    n246 = Multiply(x=w389, y=w378) -> (x*y=→"Dp2_d (Mavg)":fxp<+/-,64,41>)
  }
  n247 = while "Omega_p1 (Mavg)" {
    tunnel: w8 -> [w447]
    shift-right: [w445] -> _
    shift-left: w7 -> [w450]
    shift-right: [w444] -> _
    shift-left: w6 -> [w446]
    shift-right: [w443] -> _
    shift-left: _ -> [w442]
    tunnel: w5 -> [w440]
    stop <- FALSE stop-if-true
    w434 = fxp<+/-,27,3> 3.1415926814079285  # pi
    w433 = fxp<+/-,32,0> 0.3183098859153688  # L/2/pi
    n248 = call "Tick Count5"() -> ("Tick Count(uSec)"=w451:u32)
    n249 = Index Array(array=w450, index=0) -> (element=w449:u32)
    n250 = Index Array(array=w446, index=0) -> (element=w448:i32)
    n251 = Multiply(x=w447, y=w440) -> (x*y=w453:i32)
    n252 = Add(x=w453, y=w449) -> (x+y=w452:u32)
    n253 = Greater Or Equal?(x=w451, y=w452) -> (x >= y?=w441:bool)
    n254 = case shown="True" w441 {
      tunnel: w451 -> [_ w474]
      tunnel: w447 -> [_ w471]
      tunnel: w450 -> [w458 w473]
      tunnel: w449 -> [_ w472]
      tunnel: w448 -> [_ w468]
      tunnel: w446 -> [w457 w470]
      tunnel: [w456 w466] -> w443
      tunnel: [w458 w465] -> w445
      tunnel: [w457 w464] -> w444
      tunnel: w442 -> [w456 _]
      frame False {
      }
      frame True {
        n255 = local read "Encoder Position_p1"() -> (w467:i32)
        n256 = Subtract(x=w474, y=w472) -> (x-y=w475:u32)
        n257 = Subtract(x=w467, y=w468) -> (x-y=w460:i32)
        n258 = Insert Into Array(array=w473, new element=w474) -> (w477:u32[])  [unwired: 1 in]
        n259 = Insert Into Array(array=w470, index=w471, new element=w467) -> (w478:i32[])
        n260 = To Fixed-Point(number=w475) -> (fixed-point=w462:fxp<+,32,32>)  [unwired: 1 in]
        n261 = Multiply(x=w460, y=2500) -> (x*y=w461:i32)
        n262 = To Fixed-Point(number=w461) -> (fixed-point=w469:fxp<+/-,32,32>)  [unwired: 1 in]
        n263 = Delete From Array(array=w477, length=1, index=0) -> (array with subset deleted=w465:u32[])  [unwired: 1 out]
        n264 = Delete From Array(array=w478, length=1, index=0) -> (array with subset deleted=w464:i32[])  [unwired: 1 out]
        n265 = Divide(x=w469, y=w462) -> (x/y=w466:fxp<+/-,64,32>)
      }
    }
    n266 = local read "Belt_in_p"() -> (w438:fxp<+/-,6,6>)
    n267 = local read "Belt_out_p"() -> (w437:fxp<+/-,7,7>)
    n268 = Multiply(x=w434, y=w443) -> (x*y=w439:fxp<+/-,64,35>)
    n269 = Multiply(x=w433, y=w438) -> (x*y=w436:fxp<+/-,38,6>)
    n270 = Multiply(x=fxp<+/-,2,2> 1.0 ("f"), y=w439) -> (x*y=w432:fxp<+/-,64,37>)
    "omega_p1 (Mavg)" <- w432
    n271 = Divide(x=w436, y=w437) -> (x/y=w431:fxp<+/-,45,6>)
    n272 = Multiply(x=w431, y=w432) -> (x*y=→"Dp1_d (Mavg)":fxp<+/-,64,42>)
  }
  n273 = Merge Errors(w11, w10) -> (w12:errorcluster)
  n274 = xnode "FPGA I/O Node"("error in"=w12, "Mod6/Start"=TRUE) -> ("error out"=w16:errorcluster)  [unwired: 1 in, 1 out]
  n275 = while "PID force controller_p" {
    shift-right: [w485] -> _
    shift-left: _ -> [w484]
    stop <- FALSE stop-if-true
    n276 = local read "Force_p"() -> (w497:fxp<+/-,32,10>)
    n277 = local read "fpt_d"() -> (w493:fxp<+/-,36,18>)
    n278 = local read "Fr_p"() -> (w498:fxp<+/-,32,10>)
    n279 = Subtract(x=w498, y=w497) -> (x-y=w495:fxp<+/-,33,11>)
    "fp_tilde" <- w495
    n280 = local read "fpt_i"() -> (w489:fxp<+/-,34,18>)
    n281 = Multiply(x="Kp_p", y=w495) -> (x*y=w491:fxp<+/-,64,23>)
    n282 = Multiply(x="Kd_p", y=w493) -> (x*y=w492:fxp<+/-,64,27>)
    n283 = Absolute Value(x=w495) -> (abs(x)=w504:fxp<+,32,10>)
    n284 = Add(x=w491, y=w492) -> (x+y=w487:fxp<+/-,64,28>)
    n285 = Multiply(x="Ki_p", y=w489) -> (x*y=w488:fxp<+/-,64,27>)
    n286 = call "Tick Count7"() -> ("Tick Count(uSec)"=w485:u32)
    n287 = Add(x=w487, y=w488) -> (x+y=w486:fxp<+/-,64,29>)
    n288 = Greater?(x=w504, y="fp_tolorance") -> (0:w501:bool)
    n289 = Subtract(x=w485, y=w484) -> (x-y=w483:u32)
    n290 = Divide(x=u32 1000, y=w483) -> (x/y=→"PID (kHz)":fxp<+/-,20,7>)
    n291 = Select(t=w486, s=w501, f=fxp<+,1,1> 0.0) -> (s? t:f=→"Fp_PID":fxp<+/-,64,29>)
  }
  n292 = while "Protection" {
    stop <- FALSE stop-if-true
    n293 = local read "Force_p"() -> (w509:fxp<+/-,32,10>)
    n294 = Absolute Value(x=w509) -> (abs(x)=w508:fxp<+,32,10>)
    n295 = Greater?(x=w508, y="force_lim") -> (0:w506:bool)
    n296 = case shown="True" w506 {
      frame False {
      }
      frame True {
        n297 = local write "Stop motor_p"(TRUE ("Stop motor_p")) -> ()
      }
    }
  }
  n298 = while "ft_d" {
    stop <- FALSE stop-if-true
    n299 = local read "Dp_error_dd"() -> (w517:fxp<+/-,36,16>)
    n300 = local read "Dp_error_d"() -> (w519:fxp<+/-,33,8>)
    n301 = local read "Kv_p"() -> (w520:fxp<+/-,26,7>)
    n302 = local read "Bv_p"() -> (w518:fxp<+/-,22,8>)
    n303 = Multiply(x=w519, y=w520) -> (x*y=w515:fxp<+/-,59,15>)
    n304 = Multiply(x=w517, y=w518) -> (x*y=w516:fxp<+/-,58,24>)
    n305 = local read "Force_p"() -> (w513:fxp<+/-,32,10>)
    n306 = Add(x=w515, y=w516) -> (x+y=w514:fxp<+/-,64,24>)
    n307 = Subtract(x=w514, y=w513) -> (x-y=→"fpt_d":fxp<+/-,64,25>)
  }
  n308 = while "Derivative" {
    stop <- FALSE stop-if-true
    n309 = local read "Dpr_sin_dd"() -> (w529:fxp<+/-,35,20>)
    n310 = local read "Dpr_sin_d"() -> (w531:fxp<+/-,33,15>)
    n311 = local read "Stop motor_p"() -> (w527:bool)
    n312 = local read "Dp_error"() -> (w532:fxp<+/-,22,7>)
    n313 = local read "Dp_dd"() -> (w530:fxp<+/-,36,25>)
    n314 = Subtract(x=w531, y=w532) -> (x-y=w524:fxp<+/-,34,16>)
    n315 = Subtract(x=w529, y=w530) -> (x-y=w528:fxp<+/-,41,26>)
    n316 = Select(t=fxp<+,1,1> 0.0, s=w527, f=w524) -> (s? t:f=→"Dp_error_d":fxp<+/-,34,16>)
    n317 = Select(t=fxp<+/-,41,26> 0.0, s=w527, f=w528) -> (s? t:f=→"Dp_error_dd":fxp<+/-,41,26>)
  }
  n318 = while "Omega_p(T method)" {
    shift-right: [w564] -> _
    shift-left: _ -> [w562]
    shift-right: [w545] -> _
    shift-left: _ -> [w563]
    shift-right: [w560] -> _
    shift-left: _ -> [w561]
    shift-right: [w538] -> _
    shift-left: _ -> [w537]
    shift-right: [w533] -> _
    shift-left: _ -> [w535]
    shift-right: [w541] -> _
    shift-left: _ -> [w540]
    stop <- FALSE stop-if-true
    w552 = fxp<+/-,32,0> 0.3183098859153688  # L/2/pi
    w557 = fxp<+/-,32,0> 0.3183098859153688  # L/2/pi
    n319 = local read "Encoder Position_p1"() -> (w564:i32)
    n320 = local read "Encoder Position_p2"() -> (w538:i32)
    n321 = call "Tick Count4"() -> ("Tick Count(Ticks)"=w539:u32)
    n322 = call "omega_sub_Encoder_800ppr.vi"("mt0"="mt0_p1", "omega_pre"=w563, "ticks_m_pre"=w561, "ticks"=w539, "count_pre"=w562, "count"=w564) -> ("ticks_m"=w560:u32, "mt"=→"mt_omega_p1":u32, "omega"=w545:fxp<+/-,36,13>)  [unwired: 3 in]
    "omega_p1 (T)" <- w545
    n323 = call "omega_sub_Encoder_4096ppr.vi"("mt0"="mt0_p2", "omega_pre"=w535, "ticks_m_pre"=w540, "ticks"=w539, "count_pre"=w537, "count"=w538) -> ("ticks_m"=w541:u32, "mt"=→"mt_omega_p2":u32, "omega"=w533:fxp<+/-,36,13>)  [unwired: 3 in]
    n324 = local read "Mag. factor_p"() -> (w553:fxp<+/-,20,3>)
    n325 = local read "Belt_in_p"() -> (w550:fxp<+/-,6,6>)
    n326 = local read "Belt_out_p"() -> (w549:fxp<+/-,7,7>)
    n327 = Multiply(x=w557, y="Belt_in_p") -> (x*y=w555:fxp<+/-,38,6>)
    n328 = Multiply(x=w552, y=w550) -> (x*y=w551:fxp<+/-,38,6>)
    n329 = Divide(x=w555, y="Belt_out_p") -> (x/y=w546:fxp<+/-,20,1>)
    n330 = Divide(x=w533, y=w553) -> (x/y=w534:fxp<+/-,57,31>)
    "omega_p2 (T)" <- w534
    n331 = Divide(x=w551, y=w549) -> (x/y=w544:fxp<+/-,45,6>)
    n332 = Multiply(x=w544, y=w534) -> (x*y=→"Dp2_d (T)":fxp<+/-,36,13>)
    n333 = Multiply(x=w546, y=w545) -> (x*y=→"Dp1_d (T)":fxp<+/-,36,13>)
  }
  n334 = while {
    tunnel: [w565] -> w9
    shift-right: [w589] -> _
    shift-left: _ -> [w590]
    tunnel: w16 -> [w585]
    shift-right: [w581] -> _
    shift-left: _ -> [w582]
    shift-right: [w577] -> _
    shift-left: _ -> [w576]
    shift-right: [w576] -> _
    shift-left: _ -> [w575]
    shift-right: [w575] -> _
    shift-left: _ -> [w574]
    shift-right: [w574] -> _
    shift-left: _ -> [w573]
    shift-right: [w573] -> _
    shift-left: _ -> [w572]
    shift-right: [w572] -> _
    shift-left: _ -> [w571]
    shift-right: [w571] -> _
    shift-left: _ -> [w570]
    stop <- w584 stop-if-true
    w579 = fxp<+,20,2> 2.115001678466797  # Gage Factor
    n335 = xnode "FPGA I/O Node"("error in"=w585) -> ("error out"=w565:errorcluster, "Mod6/AI3"=w580:fxp<+/-,24,-4>)  [unwired: 1 in, 1 out]
    n336 = Select(t=w580, s="Strain gage reset_p", f=w582) -> (s? t:f=w581:fxp<+/-,24,-4>)
    n337 = Or(x="Stop (Strain)", y=w565) -> (x .or. y?=w584:bool)
    n338 = Subtract(x=w580, y=w581) -> (x-y=w578:fxp<+/-,30,-3>)
    "Mod6/AI3" <- w578
    n339 = Multiply(x=w579, y=w578) -> (x*y=w577:fxp<+/-,50,-1>)
    "Raw Strain_p" <- w577
    n340 = call "average_v2.vi"("Numeric 8"=w570, "Numeric"=w577, "Numeric 7"=w571, "Numeric 2"=w576, "Numeric 6"=w572, "Numeric 5"=w573, "Numeric 4"=w574, "Numeric 3"=w575) -> ("Mean (8pt)"=w569:fxp<+/-,32,4>)  [unwired: 1 in, 2 out]
    "Strain_p (Avg8)" <- w569
    n341 = call "Tick Count"() -> ("Tick Count(uSec)"=w589:u32)
    n342 = xnode "Butterworth Filter"("input data"=w569, "scaled coefficients"="Strain_p Avg.8 coeff.") -> ("output data"=→"Strain_p (Avg8 w. f)":fxp<+/-,36,8>)  [unwired: 1 in]
    n343 = Subtract(x=w589, y=w590) -> (x-y=w588:fxp<+/-,32,16>)
    n344 = Divide(x=fxp<+,7,10> 1000.0, y=w588) -> (x/y=→"Loop rate (kHz)":fxp<+/-,40,27>)
  }
  n345 = while {
    stop <- FALSE stop-if-true
    n346 = local read "omega_p1 (Mavg)"() -> (w606:fxp<+/-,36,14>)
    n347 = local read "Dp1_d (Mavg)"() -> (w602:fxp<+/-,36,14>)
    n348 = call "Loop Timer2"("Count(uSec)"="Mavg f loop(uSec)") -> ()  [unwired: 1 out]
    n349 = xnode "Butterworth Filter"("input data"=w606, "scaled coefficients"="omega_P(Mavg) coeff.") -> ("output data"=→"omega_p (Mavg w. f)":fxp<+/-,36,18>)  [unwired: 1 in]
    n350 = xnode "Butterworth Filter"("input data"=w602, "scaled coefficients"="Dp_d (Mavg) coeff.") -> ("output data"=→"Dp_d (Mavg w. f.)":fxp<+/-,36,18>)  [unwired: 1 in]
  }
  n351 = while "Quadrature drive_p" {
    stop <- FALSE stop-if-true
    n352 = local read "Drive mode"() -> (w624:i16)
    n353 = case shown="2" w624 {
      tunnel: [w634 w635 w636] -> w623
      frame 0, Default {
        # "Backward"
        n354 = local read "Fp_PID"() -> (w634:fxp<+/-,36,16>)
      }
      frame 1 {
        # "Forward"
        n355 = local read "Fr_p"() -> (w635:fxp<+/-,32,10>)
      }
      frame 2 {
        # "Imp"
        n356 = local read "Fp_PID"() -> (w636:fxp<+/-,36,16>)
      }
    }
    n357 = local read "dFp_PID"() -> (w627:fxp<+/-,36,18>)
    n358 = local read "omega_p (rad/s)"() -> (w631:fxp<+/-,36,13>)
    n359 = Select(t=w627, s="dFp_add", f=fxp<+,1,1> 0.0) -> (s? t:f=w630:fxp<+/-,36,18>)
    n360 = call "Oriental_step_motor_PKP225.vi"("F_Threshold"="F_Threshold_p", "dFmr"=w630, "omega"=w631, "Fmr"=w623) -> ("vq_F"=→"vq_p_F":fxp<+/-,36,9>, "vd_F"=→"vd_p_F":fxp<+/-,36,9>)  [unwired: 6 in]
  }
  n361 = xnode "FPGA I/O Node"("error in"=w9, "Mod6/Stop"=TRUE) -> ()  [unwired: 1 in, 2 out]
